vi "Close Hardware.vi"(8 "error in (no error)":errorcluster, 11 "Inst.TSL210 in":refnum<class "Inst.TSL210.lvclass">) -> (0 "error out":errorcluster, 3 "Inst.TSL210 out":refnum<class "Inst.TSL210.lvclass">)   [LabVIEW 2019, in "Inst.TSL210.lvclass"]
uses:
  Inst.TSL210.lvclass
  <userlib>/LevyLab/Instrument Framework/Instrument Types/VSource/Instrument.VSource.lvclass
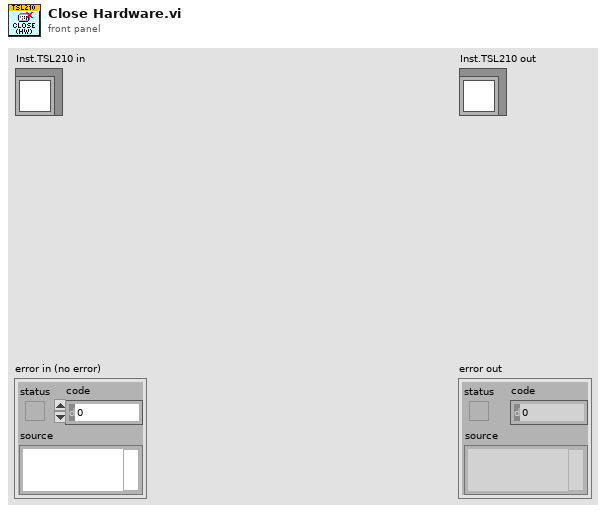
[diagram p1: front panel]
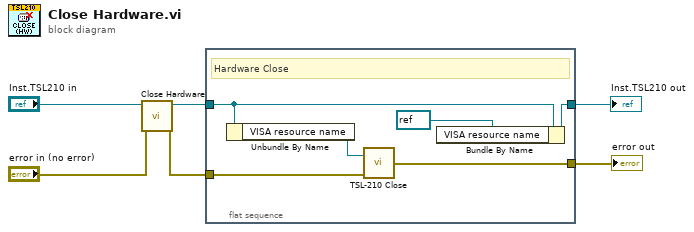
[diagram p0: block diagram]
diagram:
  n1 = call-parent "Close Hardware.vi"("error in (no error)"="error in (no error)", "Instrument in"="Inst.TSL210 in") -> ("error out"=w4:errorcluster, "Instrument out"=w3:refnum<class "Inst.TSL210.lvclass">)  [unwired: 8 in]
  n2 = flat-sequence {
    tunnel: w4 -> [w8]
    tunnel: w3 -> [w12]
    tunnel: [w11] -> w2
    tunnel: [w7] -> w1
    frame #0 {
      # "Hardware Close"
      n3 = Unbundle By Name(w12) -> ("VISA resource name"=w9:refnum<visa-resource-name>)
      n4 = call "TSL-210 Close.vi"("error in (no error)"=w8, "VISA Session"=w9) -> ("error out"=w7:errorcluster)
      n5 = Bundle By Name(cluster=w12, "VISA resource name"=refnum<visa-resource-name> refnum) -> (w11:refnum<class "Inst.TSL210.lvclass">)
    }
  }
  "error out" <- w1
  "Inst.TSL210 out" <- w2
